vi "toml_remove_section.vi"(4 "vi":refnum<vi>, 7 "section":string, 8 "error in (no error)":errorcluster, 11 "path in":path) -> (0 "error out":errorcluster, 2 "section exists":bool, 3 "path out":path)   [LabVIEW 2017]
uses:
  <vilib>/Utility/error.llb/Clear Errors.vi
  toml_lock_obtain.vi
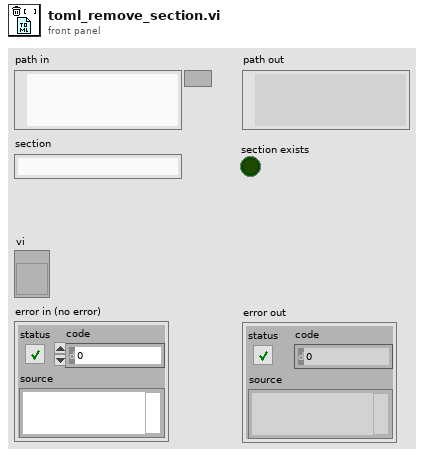
[diagram p1: front panel]
types:
  T1 = enum16{"open", "replace", "create", "open or create", "replace or create", "replace or create with confirmation"}
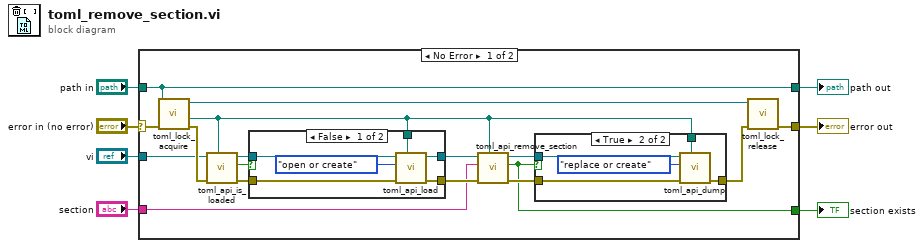
[diagram p0: block diagram]
diagram:
  n1 = case shown="No Error" "error in (no error)" {
    selector: "error in (no error)" -> [w23 w39]
    tunnel: [w22 w39] -> w6
    tunnel: "vi" -> [w16 _]
    tunnel: "path in" -> [w21 w40]
    tunnel: [w21 w40] -> w3
    tunnel: "section" -> [w12 _]
    tunnel: [w8 _] -> w1
    frame No Error {
      n2 = call "toml_lock_acquire.vi"("error in (no error)"=w23, "path in"=w21) -> ("error out"=w17:errorcluster, "resolved path"=w13:path, "lock"=w24:refnum<queue>)  [unwired: 7 in]
      n3 = call "toml_api_is_loaded.vi"("resolved path"=w13, "error in (no error)"=w17, "vi in"=w16) -> ("error out"=w19:errorcluster, "file loaded"=w20:bool, "vi out"=w18:refnum<vi>)  [unwired: 5 in, 1 out]
      n4 = case shown="False" w20 {
        tunnel: w19 -> [w30 w32]
        tunnel: [w29 w32] -> w15
        tunnel: w13 -> [w26 _]
        tunnel: w18 -> [w28 w31]
        tunnel: [w27 w31] -> w14
        frame False {
          n5 = call "toml_api_load.vi"("resolved path"=w26, "error in (no error)"=w30, "operation"=T1."open or create" ("operation (open or create)"), "vi in"=w28) -> ("error out"=w29:errorcluster, "vi out"=w27:refnum<vi>)  [unwired: 5 in, 1 out]
        }
        frame True {
        }
      }
      n6 = call "toml_api_remove_section.vi"("resolved path"=w13, "error in (no error)"=w15, "section"=w12, "vi in"=w14) -> ("error out"=w11:errorcluster, "section exists"=w8:bool, "vi out"=w10:refnum<vi>)  [unwired: 5 in]
      n7 = case shown="True" w8 {
        tunnel: w13 -> [_ w36]
        tunnel: w11 -> [w33 w38]
        tunnel: w10 -> [_ w37]
        tunnel: [w33 w34] -> w9
        frame False {
        }
        frame True {
          n8 = call "toml_api_dump.vi"("resolved path"=w36, "error in (no error)"=w38, "operation (open or create)"=T1."replace or create", "vi in"=w37) -> ("error out"=w34:errorcluster)  [unwired: 5 in, 2 out]
        }
      }
      n9 = call "toml_lock_release.vi"("error in (no error)"=w9, "lock"=w24) -> ("error out"=w22:errorcluster)  [unwired: 9 in]
    }
    frame Error {
    }
  }
  "error out" <- w6
  "path out" <- w3
  "section exists" <- w1
